vi "MENU - Parse Item Tag.vi"(0 "reference in":refnum<class "Generic Utilities.lvclass">, 5 "error in (no error)":errorcluster, 6 "Item Tag":string) -> (9 "Tag 2":string, 11 "Tag 1":string, 13 "Case":string, 14 "reference out":refnum<class "Generic Utilities.lvclass">, 19 "error out":errorcluster)   [LabVIEW 2020, in "Generic Utilities.lvclass"]
uses:
  Generic Utilities.lvclass
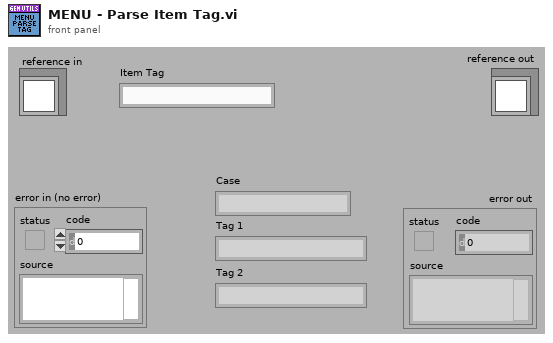
[diagram p1: front panel]
types:
  T1 = typedef "Generic Utilities.lvclass/ObjectAttributes.ctl" = cluster{"GUI Parameters":T2, "State Machine Control":cluster{"Timeout":i32, "State Queue":string[], "State History":string[], "State History Length":i32}, "Logging File Path":path, "OBJ not a refnum?":bool, "Timer Start":timestamp, "FP Refnums":T3}
  T2 = typedef "Generic Utilities.lvclass/GUI Parameters.ctl" = cluster{"Application Name":string, "GUI VI Ref":refnum<vi>, "Close Panel?":bool, "Message Window ref":refnum<vi>, "Version #":string}
  T3 = typedef "Generic Utilities.lvclass/FP Refnums.ctl" = cluster{"Panel refnum":refnum<vi>, "Control Labels":string[], "Refnums":refnum<vi>[]}
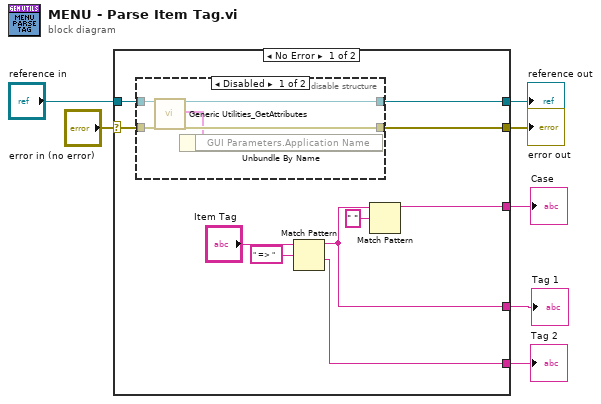
[diagram p0: block diagram]
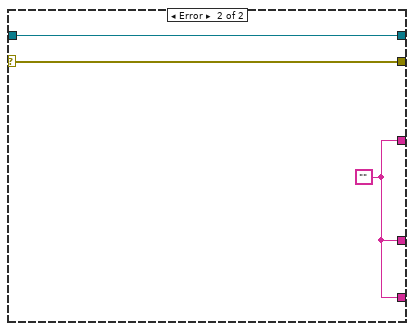
[diagram p3: hidden frame]
diagram:
  n1 = case shown="No Error" "error in (no error)" {
    selector: "error in (no error)" -> [w17 w27]
    tunnel: [w16 w27] -> w6
    tunnel: [w15 w26] -> w4
    tunnel: "reference in" -> [w14 w26]
    tunnel: [w8 w25] -> w3
    tunnel: [w11 w25] -> w2
    tunnel: [w10 w25] -> w1
    frame No Error {
      n2 = disable-structure shown="Disabled" {
        disable-tunnel: w17 -> [w22 w23]
        disable-tunnel: [w21 w23] -> w16
        disable-tunnel: [w20 w24] -> w15
        disable-tunnel: w14 -> [w19 w24]
        frame Disabled {
          n3 = call "Generic Utilities_GetAttributes.vi"("reference in"=w19, "error in (no error)"=w22) -> ("reference out"=w20:refnum<class "Generic Utilities.lvclass">, "attributes"=w18:T1, "error out"=w21:errorcluster)  [unwired: 14 in, 1 out]
          n4 = Unbundle By Name(w18) -> ()  [unwired: 1 out]
        }
        frame Enabled {
        }
      }
      n5 = Match Pattern(string="Item Tag", regular expression=" => " ("string")) -> (before substring=w10:string, after substring=w11:string)  [unwired: 1 in, 2 out]
      n6 = Match Pattern(string=w10, regular expression=" ") -> (before substring=w8:string)  [unwired: 1 in, 3 out]
    }
    frame Error {
      w25 = ""
    }
  }
  "error out" <- w6
  "reference out" <- w4
  "Tag 2" <- w2
  "Case" <- w3
  "Tag 1" <- w1
